vi "vision 2.vi"() -> ()   [LabVIEW 2012]
uses:
  <vilib>/event_ctls.llb/lveventtype.ctl
  <vilib>/vision/driver/IMAQdx.llb/IMAQdx Buffer Number Mode.ctl
  <vilib>/vision/driver/NI_Vision_Acquisition_Software.lvlib
  <vilib>/vision/NI_Vision_Development_Module.lvlib
panel:
  out "Image":T1(plugin-control)
  in  "stop":bool
  in  "Slide":dbl(slide)=100.0 scale=10.0..1000.0
  out "?":T2(array[cluster]) {"Bounding Box"."y" format="%.2f"; "Bounding Box"."x" format="%.2f"; "Position"."y" format="%.2f"; "Position"."x" format="%.2f"; "Score" format="%.2f"; "Escala" format="%.2f"; "Angle" format="%.2f"}
  out "Type":T3
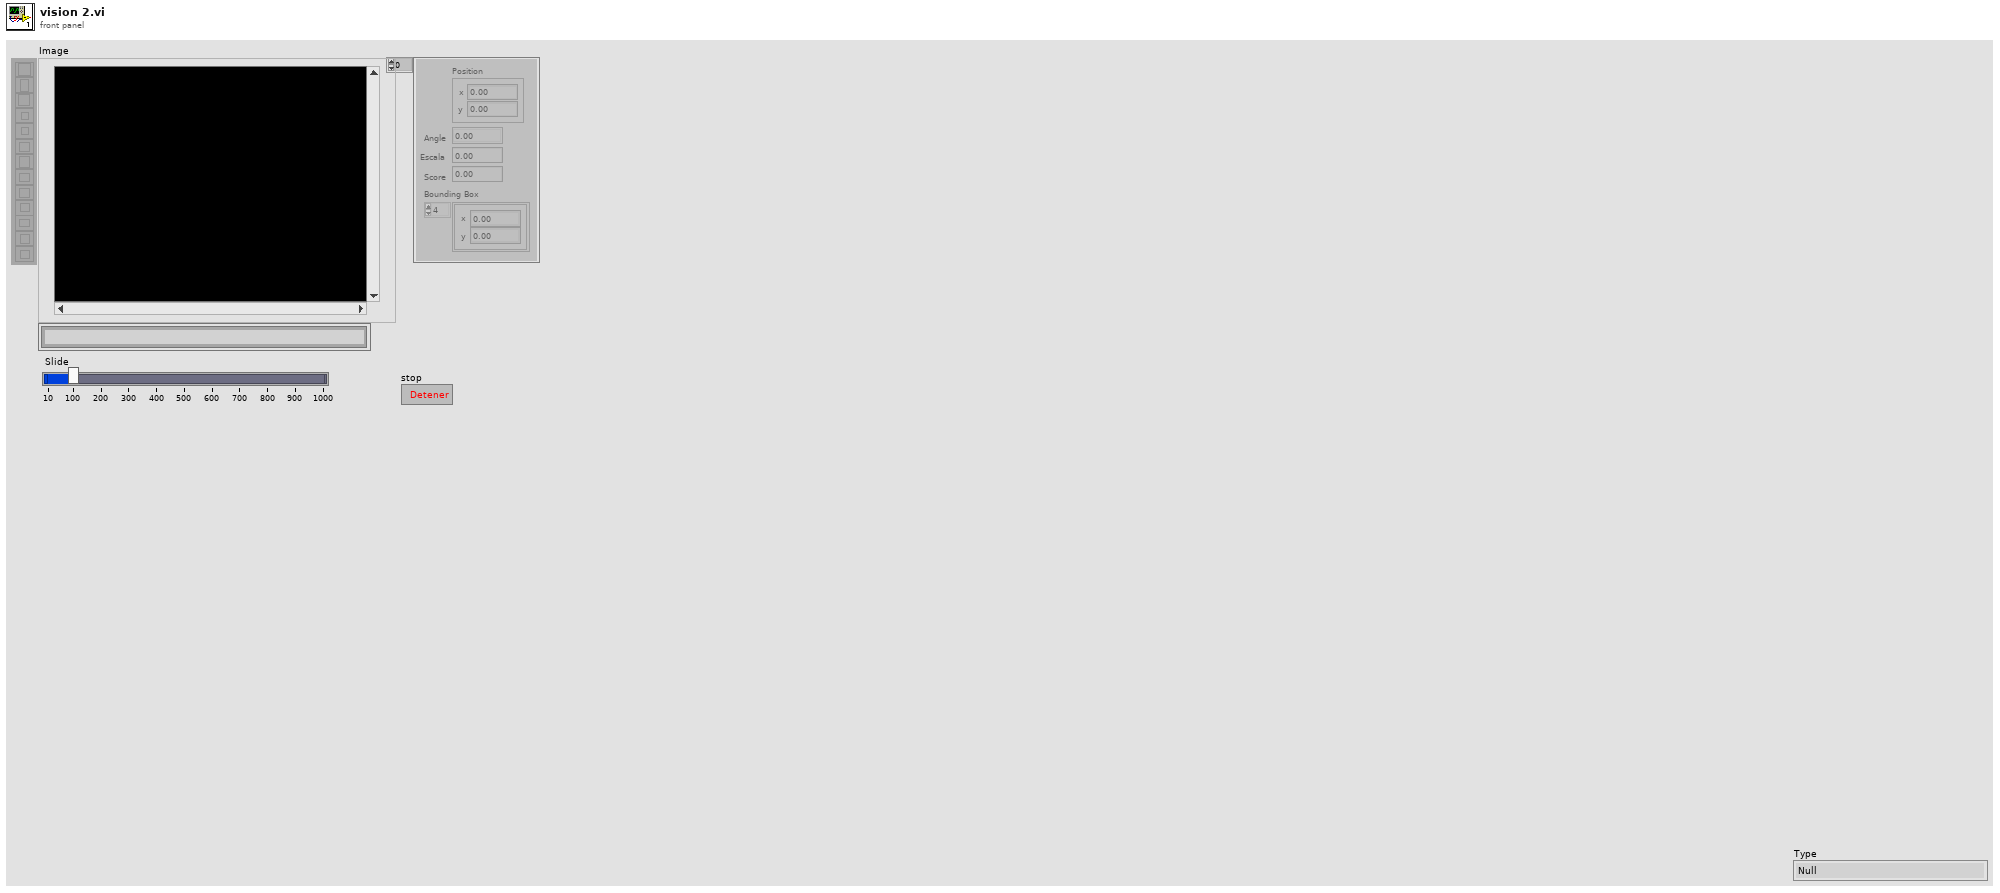
[diagram p1: front panel]
types:
  T1 = typedef "IMAQ Image.ctl" = refnum<image>
  T2 = cluster{"Position":cluster{"x":sgl, "y":sgl}, "Angle":sgl, "Escala":sgl, "Score":sgl, "Bounding Box":cluster{"x":sgl, "y":sgl}[]}[]
  T3 = typedef "lveventtype.ctl" = enum32{"Null", "Timeout", "Annotation Menu Selection", "Annotation Menu Selection?", "App Instance Close", "App Instance Close?", "Autoscale Range Change", "Cell Edit", "Cell Edit?", "Cursor Grab", "Cursor Grab?", "Cursor Menu Selection", "Cursor Menu Selection?", "Cursor Move", "Cursor Release", "Data Change", "Direction Change", "Display State Change", "Drag Ended", "Drag Enter", "Drag Leave", "Drag Over", "Drag Source Update", "Drag Starting", "Drag Starting?", "Drop", "Exec State Change", "Key Down", "Key Down?", "Key Repeat", "Key Repeat?", "Key Up", "Listbox Double Click", "Menu Activation?", "Menu Selection (App)", "Menu Selection? (App)", "Menu Selection (User)", "Mouse Down", "Mouse Down?", "Mouse Enter", "Mouse Leave", "Mouse Move", "Mouse Up", "NI Security User Change (App)", "Pane Size", "Panel Close", "Panel Close?", "Panel Resize", "Plot Attribute Change", "Scale Range Change", "Shortcut Menu Activation?", "Shortcut Menu Selection (App)", "Shortcut Menu Selection? (App)", "Shortcut Menu Selection (User)", "Tree Double Click", "Tree Drag", "Tree Drag?", "Tree Drop", "Tree Drop?", "Tree Item Close", "Tree Item Close?", "Tree Item Open", "Tree Item Open?", "Value Change"}
  T4 = typedef "Image Type" = u32
  T5 = typedef "IMAQdx.ctl" = refnum<k21>
  T6 = typedef "NI_Vision_Acquisition_Software.lvlib/IMAQdx Buffer Number Mode.ctl" = enum32{"Next", "Last", "Buffer Number"}
  T7 = typedef "ROI Descriptor" = cluster{"Global Rectangle":i32[], "Contours":cluster{"ID":enum32{"External", "Internal"}, "Type":u32, "Coordinates":i32[]}[]}
  T8 = cluster{"Position":cluster{"x":sgl, "y":sgl}, "Angle":sgl, "Scale":sgl, "Score":sgl, "Bounding Box":cluster{"x":sgl, "y":sgl}[]}[]
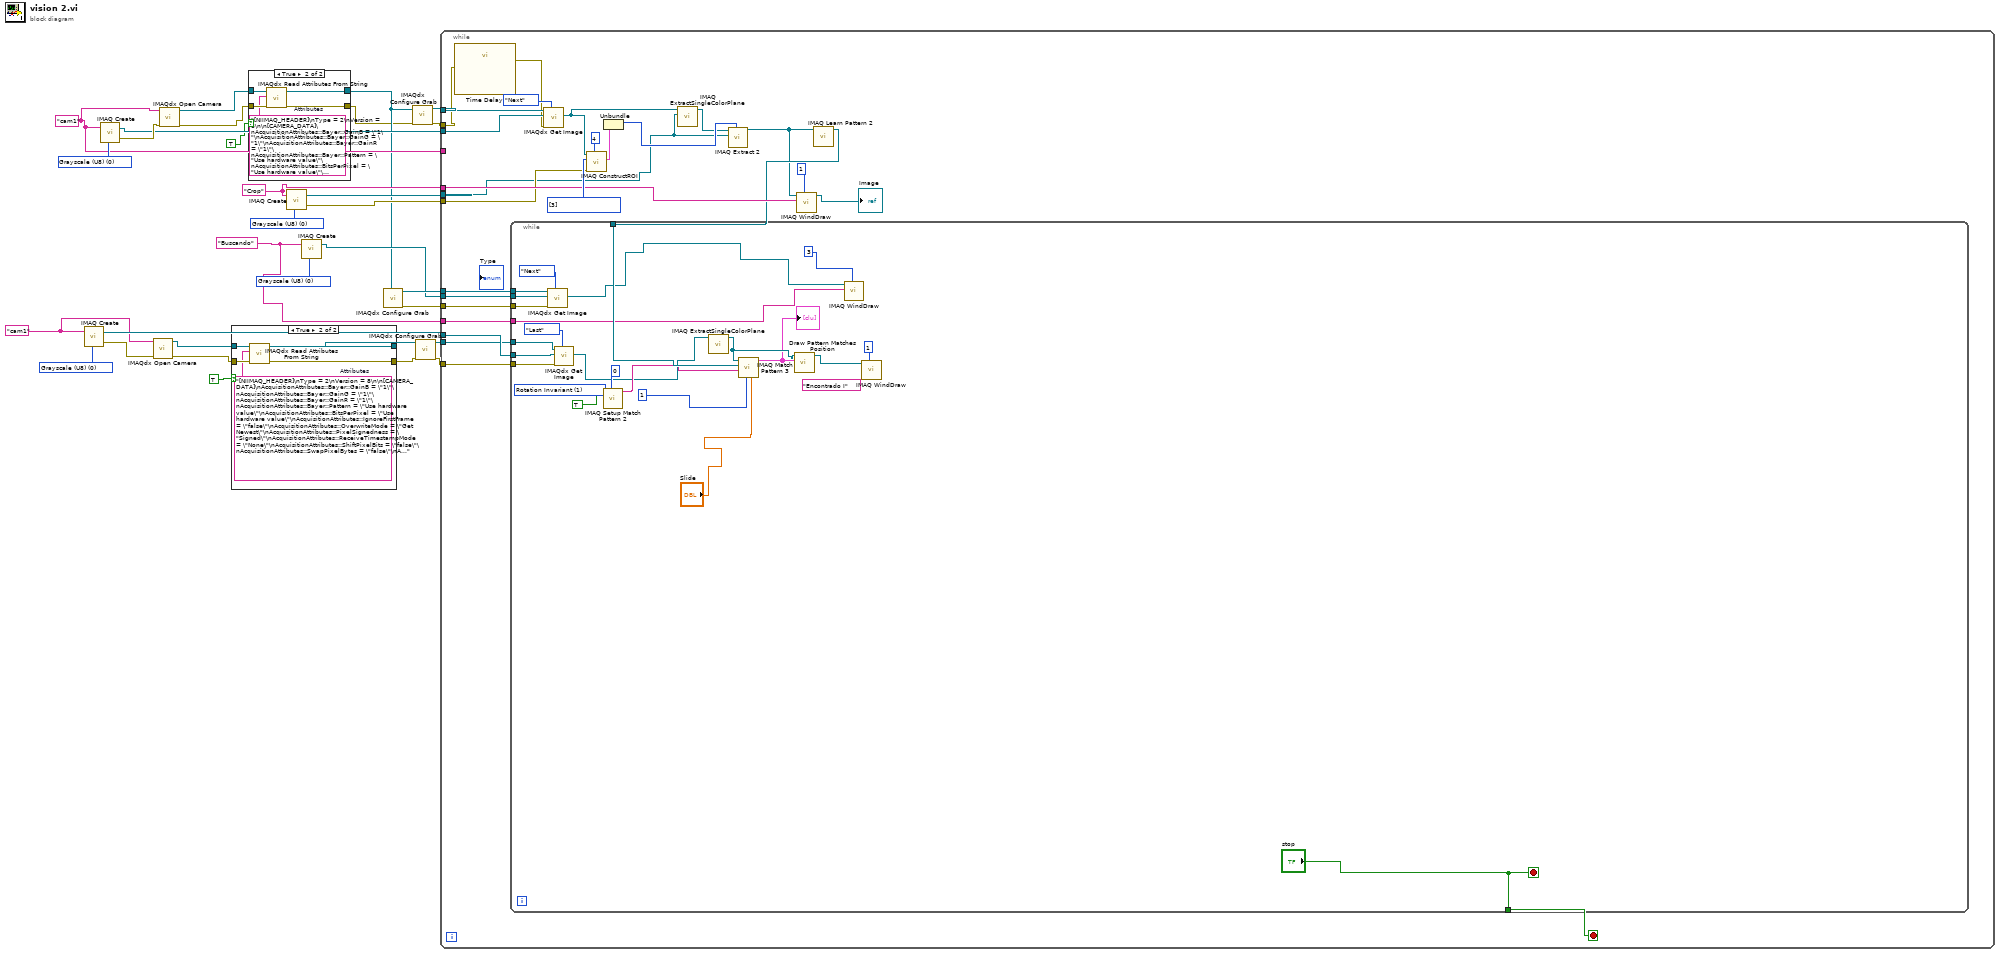
[diagram p0: block diagram]
diagram:
  w12 = "cam1" ("Image Name")
  w1 = "Buscando" ("Image Name")
  w21 = "Crop" ("Image Name")
  w23 = "cam1" ("Image Name")
  w28 = T4 0 items=["Grayscale (U8)", "Grayscale (I16)", "Grayscale (SGL)", "Complex (CSG)", "RGB (U32)", "HSL (U32)", "RGB (U64)", "Grayscale (U16)"] ("Image Type")
  w29 = T4 0 items=["Grayscale (U8)", "Grayscale (I16)", "Grayscale (SGL)", "Complex (CSG)", "RGB (U32)", "HSL (U32)", "RGB (U64)", "Grayscale (U16)"] ("Image Type")
  w30 = T4 0 items=["Grayscale (U8)", "Grayscale (I16)", "Grayscale (SGL)", "Complex (CSG)", "RGB (U32)", "HSL (U32)", "RGB (U64)", "Grayscale (U16)"] ("Image Type")
  w31 = T4 0 items=["Grayscale (U8)", "Grayscale (I16)", "Grayscale (SGL)", "Complex (CSG)", "RGB (U32)", "HSL (U32)", "RGB (U64)", "Grayscale (U16)"] ("Image Type")
  n1 = call "IMAQ Create"("Image Name"=w12, "Image Type"=w28) -> ("New Image"=w18:T1, "error out"=w26:errorcluster)  [unwired: 3 in]
  n2 = call "IMAQ Create"("Image Name"=w23, "Image Type"=w31) -> ("New Image"=w22:T1, "error out"=w27:errorcluster)  [unwired: 3 in]
  n3 = call <vilib>:"IMAQdx Open Camera.vi"("error in"=w26, "Session In"=w12) -> ("error out"=w4:errorcluster, "Session Out"=w7:T5)  [unwired: 1 in, 7 out]
  n4 = call <vilib>:"IMAQdx Open Camera.vi"("error in"=w27, "Session In"=w23) -> ("error out"=w10:errorcluster, "Session Out"=w2:T5)  [unwired: 1 in, 7 out]
  n5 = case shown="True" TRUE ("Init Attributes") {
    tunnel: w7 -> [w33 w38]
    tunnel: w4 -> [w32 w37]
    tunnel: [w33 w35] -> w6
    tunnel: [w32 w34] -> w5
    frame False {
    }
    frame True {
      w36 = "[NIIMAQ_HEADER]\nType = 2\nVersion = 8\n\n[CAMERA_DATA]\nAcquisitionAttributes::Bayer::GainB = \"1\"\nAcquisitionAttributes::Bayer::GainG = \"1\"\nAcquisitionAttributes::Bayer::GainR = \"1\"\nAcquisitionAttributes::Bayer::Pattern = \"Use hardware value\"\nAcquisitionAttributes::BitsPerPixel = \"Use hardware value\"\nAcquisitionAttributes::IgnoreFirstFrame = \"false\"\nAcquisitionAttributes::OverwriteMode = \"Get Newest\"\nAcquisitionAttributes::PixelSignedness = \"Signed\"\nAcquisitionAttributes::ReceiveTimestampMode = \"None\"\nAcquisitionAttributes::ShiftPixelBits = \"false\"\nAcquisitionAttributes::SwapPixelBytes = \"false\"\nAcquisitionAttributes::Timeout = \"5000\"\nAcquisitionAttributes::VerticalMirror = \"false\"\nAcquisitionAttributes::VideoMode =\"640x480 RGB24 30.00fps\"\nCameraAttributes::BacklightCompensation::Mode = \"Manual\"\nCameraAttributes::BacklightCompensation::Value = \"true\"\nCameraAttributes::Brightness::Mode = \"Manual\"\nCameraAttributes::Brightness::Value = \"125\"\nCameraAttributes::ColorEnable::Mode = \"Manual\"\nCameraAttributes::ColorEnable::Value = \"true\"\nCameraAttributes::Contrast::Mode = \"Manual\"\nCameraAttributes::Contrast::Value = \"0.45000000000000001\"\nCameraAttributes::Exposure::Mode = \"Auto\"\nCameraAttributes::Gamma::Mode = \"Manual\"\nCameraAttributes::Gamma::Value = \"0.59999999999999998\"\nCameraAttributes::Hue::Mode = \"Manual\"\nCameraAttributes::Hue::Value = \"0\"\nCameraAttributes::Saturation::Mode = \"Manual\"\nCameraAttributes::Saturation::Value = \"165\"\nCameraAttributes::Sharpness::Mode = \"Manual\"\nCameraAttributes::Sharpness::Value = \"7\"\nCameraAttributes::WhiteBalance::Mode = \"Auto\"\nCameraAttributes::Zoom::Mode = \"Manual\"\nCameraAttributes::Zoom::Value = \"0\"\n"  # Attributes
      n6 = call <vilib>:"IMAQdx Read Attributes From String.vi"("error in"=w37, "Attributes String In"=w36, "Session In"=w38) -> ("error out"=w34:errorcluster, "Session Out"=w35:T5)  [unwired: 7 out]
    }
  }
  n7 = case shown="True" TRUE ("Init Attributes") {
    tunnel: w2 -> [w40 w45]
    tunnel: w10 -> [w39 w44]
    tunnel: [w40 w42] -> w11
    tunnel: [w39 w41] -> w9
    frame False {
    }
    frame True {
      w43 = "[NIIMAQ_HEADER]\nType = 2\nVersion = 8\n\n[CAMERA_DATA]\nAcquisitionAttributes::Bayer::GainB = \"1\"\nAcquisitionAttributes::Bayer::GainG = \"1\"\nAcquisitionAttributes::Bayer::GainR = \"1\"\nAcquisitionAttributes::Bayer::Pattern = \"Use hardware value\"\nAcquisitionAttributes::BitsPerPixel = \"Use hardware value\"\nAcquisitionAttributes::IgnoreFirstFrame = \"false\"\nAcquisitionAttributes::OverwriteMode = \"Get Newest\"\nAcquisitionAttributes::PixelSignedness = \"Signed\"\nAcquisitionAttributes::ReceiveTimestampMode = \"None\"\nAcquisitionAttributes::ShiftPixelBits = \"false\"\nAcquisitionAttributes::SwapPixelBytes = \"false\"\nAcquisitionAttributes::Timeout = \"5000\"\nAcquisitionAttributes::VerticalMirror = \"false\"\nAcquisitionAttributes::VideoMode =\"640x480 RGB24 30.00fps\"\nCameraAttributes::BacklightCompensation::Mode = \"Manual\"\nCameraAttributes::BacklightCompensation::Value = \"true\"\nCameraAttributes::Brightness::Mode = \"Manual\"\nCameraAttributes::Brightness::Value = \"125\"\nCameraAttributes::ColorEnable::Mode = \"Manual\"\nCameraAttributes::ColorEnable::Value = \"true\"\nCameraAttributes::Contrast::Mode = \"Manual\"\nCameraAttributes::Contrast::Value = \"0.45000000000000001\"\nCameraAttributes::Exposure::Mode = \"Auto\"\nCameraAttributes::Gamma::Mode = \"Manual\"\nCameraAttributes::Gamma::Value = \"0.59999999999999998\"\nCameraAttributes::Hue::Mode = \"Manual\"\nCameraAttributes::Hue::Value = \"0\"\nCameraAttributes::Saturation::Mode = \"Manual\"\nCameraAttributes::Saturation::Value = \"165\"\nCameraAttributes::Sharpness::Mode = \"Manual\"\nCameraAttributes::Sharpness::Value = \"7\"\nCameraAttributes::WhiteBalance::Mode = \"Auto\"\nCameraAttributes::Zoom::Mode = \"Manual\"\nCameraAttributes::Zoom::Value = \"0\"\n"  # Attributes
      n8 = call <vilib>:"IMAQdx Read Attributes From String.vi"("error in"=w44, "Attributes String In"=w43, "Session In"=w45) -> ("error out"=w41:errorcluster, "Session Out"=w42:T5)  [unwired: 7 out]
    }
  }
  n9 = call "IMAQ Create"("Image Name"=w21, "Image Type"=w30) -> ("New Image"=w20:T1, "error out"=w19:errorcluster)  [unwired: 3 in]
  n10 = call "IMAQ Create"("Image Name"=w1, "Image Type"=w29) -> ("New Image"=w13:T1)  [unwired: 3 in, 1 out]
  n11 = call <vilib>:"IMAQdx Configure Grab.vi"("Session In"=w11) -> ("error out"=w15:errorcluster, "Session Out"=w14:T5)  [unwired: 1 in, 8 out]
  n12 = call <vilib>:"IMAQdx Configure Grab.vi"("error in"=w9, "Session In"=w11) -> ("error out"=w24:errorcluster, "Session Out"=w25:T5)  [unwired: 8 out]
  n13 = call <vilib>:"IMAQdx Configure Grab.vi"("error in"=w5, "Session In"=w6) -> ("error out"=w17:errorcluster, "Session Out"=w16:T5)  [unwired: 8 out]
  n14 = while {
    tunnel: w25 -> [w68]
    tunnel: w24 -> [w49]
    tunnel: w23 -> [_]
    tunnel: w22 -> [w67]
    tunnel: w21 -> [w66]
    tunnel: w20 -> [w51]
    tunnel: w19 -> [w65]
    tunnel: w18 -> [w63]
    tunnel: w17 -> [w62]
    tunnel: w16 -> [w61]
    tunnel: w15 -> [w60]
    tunnel: w14 -> [w59]
    tunnel: w13 -> [w58]
    tunnel: w1 -> [w47]
    stop <- w57 stop-if-true
    w71 = u32[] [3] items=["No Selection", "Point", "Line", "Rectangle", "Oval", "Polygon", "Freehand Region", "Annulus", "Zoom", "Pan", "Broken Line", "Freehand Line", "Rotated Rectangle"] ("Tools")
    n15 = call "Time Delay"("error in (no error)"=w49) -> ("error out"=w48:errorcluster)  [unwired: 10 in]
    n16 = call <vilib>:"IMAQdx Get Image.vi"("Buffer Number Mode (Next)"=IMAQdx_Buffer_Number_Mode."Next", "error in"=w48, "Image In"=w67, "Session In"=w68) -> ("Image Out"=w52:T1)  [unwired: 4 in, 3 out]
    n17 = call "IMAQ ConstructROI"("Window Number (-1...15)"=4, "error in (no error)"=w65, "Tools"=w71, "Image"=w52) -> ("ROI Descriptor Out"=w69:T7)  [unwired: 4 in, 3 out]
    n18 = Unbundle(w69) -> ("Global Rectangle"=w55:i32[])  [unwired: 1 out]
    n19 = call "IMAQ ExtractSingleColorPlane"("Image Dst"=w51, "Image Src"=w52) -> ("Image Dst Out"=w50:T1)  [unwired: 8 in, 1 out]
    n20 = call "IMAQ Extract 2"("Optional Rectangle"=w55, "Image Dst"=w51, "Image Src"=w50) -> ("Image Dst Out"=w53:T1)  [unwired: 7 in, 1 out]
    n21 = call "IMAQ WindDraw"("Window Number (0...15)"=1, "Title"=w66, "Image"=w53) -> ("Image Out (duplicate)"=→"Image":T1)  [unwired: 7 in, 1 out]
    n22 = call "IMAQ Learn Pattern 2"("Image"=w53) -> ("Template Image Out"=w54:T1)  [unwired: 9 in, 1 out]
    n23 = while {
      tunnel: w63 -> [w94]
      tunnel: w62 -> [w93]
      tunnel: w61 -> [w92]
      tunnel: w60 -> [w91]
      tunnel: w59 -> [w90]
      tunnel: w58 -> [w89]
      tunnel: w54 -> [w87]
      tunnel: ["stop"] -> w57
      tunnel: w47 -> [w78]
      stop <- "stop" stop-if-true
      w96 = u16 1 items=["Shift Invariant", "Rotation Invariant"] ("Match Mode")
      n24 = call <vilib>:"IMAQdx Get Image.vi"("Buffer Number Mode (Next)"=IMAQdx_Buffer_Number_Mode."Next", "error in"=w91, "Image In"=w89, "Session In"=w90) -> ("Image Out"=w73:T1)  [unwired: 4 in, 3 out]
      n25 = call <vilib>:"IMAQdx Get Image.vi"("Buffer Number Mode (Next)"=IMAQdx_Buffer_Number_Mode."Last", "error in"=w93, "Image In"=w94, "Session In"=w92) -> ("Image Out"=w81:T1)  [unwired: 4 in, 3 out]
      n26 = call "IMAQ Setup Match Pattern 2"("Minimum Contrast"=0, "Subpixel Accuracy"=TRUE, "Match Mode"=w96) -> ("Match Pattern Setup Data"=w86:string)  [unwired: 7 in, 1 out]
      n27 = call "IMAQ ExtractSingleColorPlane"("Image Src"=w81) -> ("Image Dst Out"=w75:T1)  [unwired: 9 in, 1 out]
      n28 = call "IMAQ Match Pattern 3"("Minimum Match Score"="Slide", "Number of Matches Requested"=1, "Match Pattern Setup Data"=w86, "Template Image"=w87, "Image"=w75) -> ("Matches"=w74:T8)  [unwired: 4 in, 2 out]
      "?" <- w74
      n29 = call "Draw Pattern Matches Position .vi"("Matches"=w74, "Image"=w75) -> ("Image Out"=w72:T1)  [unwired: 9 in]
      n30 = call "IMAQ WindDraw"("Window Number (0...15)"=3, "Title"=w78, "Image"=w73) -> ()  [unwired: 7 in, 2 out]
      n31 = call "IMAQ WindDraw"("Window Number (0...15)"=1, "Title"="Encontrado I", "Image"=w72) -> ()  [unwired: 7 in, 2 out]
    }
  }
